vi "Create Duplicate String Indicators for Clusters.vi"(0 "UI VI Ref":refnum<vi>, 11 "error in (no error)":errorcluster) -> (4 "UI VI Ref Out":refnum<vi>, 15 "error out":errorcluster)   [LabVIEW 2021, in "Migrator.lvlib"]
uses:
  Migrator.lvlib
  Migrator Reusables/Migrator Reusables.lvlib
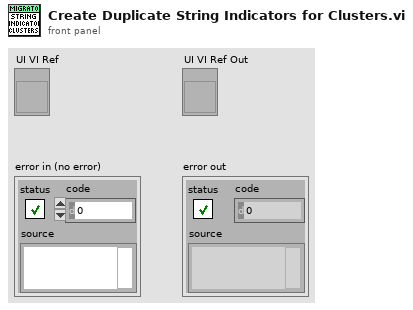
[diagram p1: front panel]
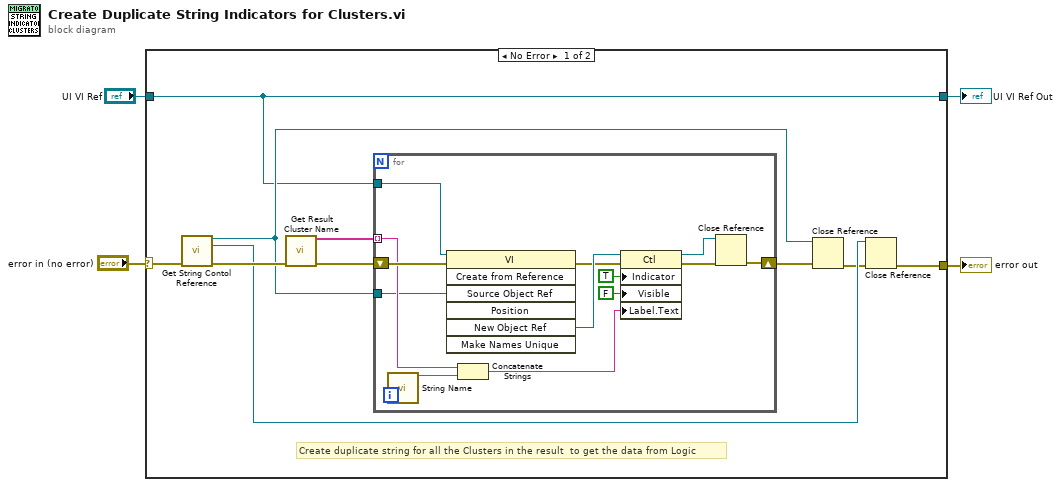
[diagram p0: block diagram]
diagram:
  n1 = case shown="No Error" "error in (no error)" {
    selector: "error in (no error)" -> [w12 w29]
    tunnel: [w6 w29] -> w4
    tunnel: "UI VI Ref" -> [w5 w28]
    tunnel: [w5 w28] -> w1
    frame No Error {
      # "Create duplicate string for all the Clusters in the result  to get the data from Logic"
      n2 = call "Get String Contol Reference.vi"("error in (no error)"=w12) -> ("String"=w10:refnum<vi>, "vi reference"=w8:refnum<vi>, "error out"=w11:errorcluster)  [unwired: 12 in]
      n3 = call "Get Result Cluster Name.vi"("error in (no error)"=w11) -> ("Control Names Out"=w13:string[], "error out"=w14:errorcluster)  [unwired: 12 in, 1 out]
      n4 = for {
        shift-right: [w15] -> w9
        shift-left: w14 -> [w27]
        tunnel: w13 -> [w20] mode=indexing
        tunnel: w5 -> [w26]
        tunnel: w10 -> [w16]
        n5 = call "String Name.vi"() -> ("Postfix"=w21:string)  [unwired: 15 in]
        n6 = invoke class="VI" method="Create from Reference"(reference=w26, error in=w27, "Source Object Ref"=w16) -> (error out=w24:errorcluster, "New Object Ref"=w25:refnum<vi>)  [unwired: 4 in, 5 out]
        n7 = Concatenate Strings(w20, w21) -> (w19:string)
        n8 = property class="Ctl"(reference=w25, error in=w24, "Indicator"=TRUE, "Visible"=FALSE, "Label.Text"=w19) -> (reference out=w17:refnum<vi>, error out=w18:errorcluster)
        n9 = Close Reference(reference=w17, error in (no error)=w18) -> (error out=w15:errorcluster)
      }
      n10 = Close Reference(reference=w10, error in (no error)=w9) -> (error out=w7:errorcluster)
      n11 = Close Reference(reference=w8, error in (no error)=w7) -> (error out=w6:errorcluster)
    }
    frame Error {
    }
  }
  "error out" <- w4
  "UI VI Ref Out" <- w1
